vi "Document VI.vi"(6 "Variant in":variant, 7 "Shift Pressed?":bool, 8 "error in (no error)":errorcluster, 10 "QD Combo Box Ref":refnum<vi>, 11 "QD Launch VI Ref":refnum<vi>) -> (0 "error out":errorcluster, 4 "Variant out":variant)   [LabVIEW 2020, in "lv_documentation.lvlib"]
doc: "Write a 1-2 sentence description of the functionality of your plugin here. Replace the \"$\" below with the character you wish to assign as the default shortcut for this plugin. Do not add any text after the 'Default Shortcut' line below.\n\nDefault Shortcut - [$]"
uses:
  lv_documentation.lvlib
panel:
  in  "Undo Name":string="Quick Drop Keyboard Shortcut"
  # "Specify the name of the Undo transaction"
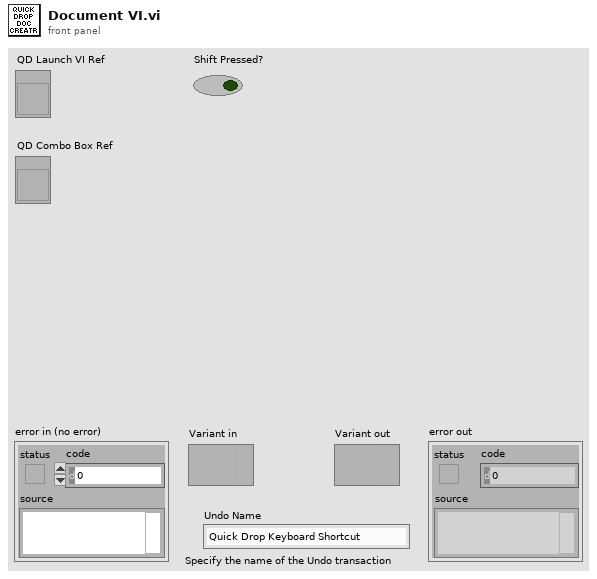
[diagram p1: front panel]
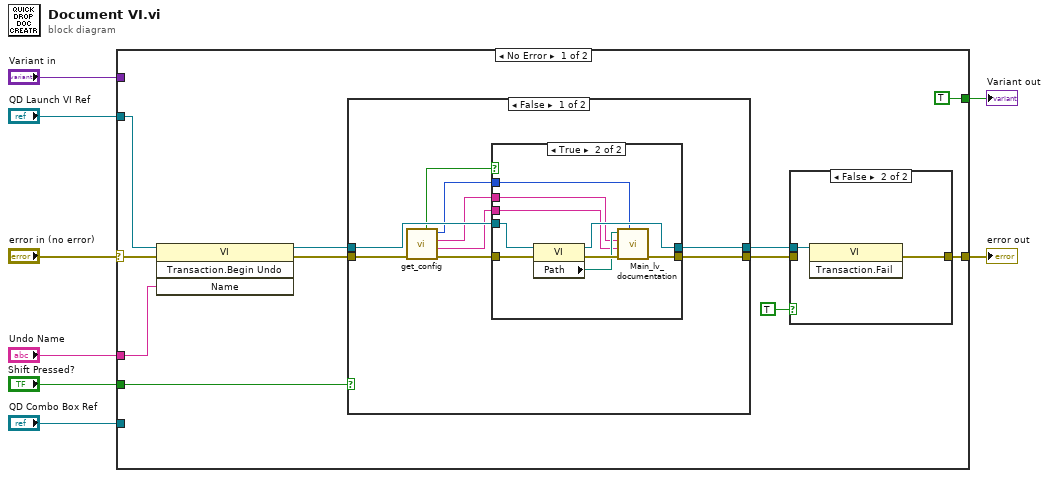
[diagram p0: block diagram]
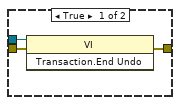
[diagram p2: hidden frame]
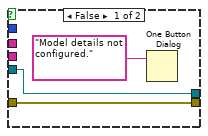
[diagram p3: hidden frame]
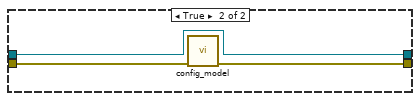
[diagram p4: hidden frame]
diagram:
  n1 = case shown="No Error" "error in (no error)" {
    selector: "error in (no error)" -> [w19 w49]
    tunnel: [w15 w49] -> w7
    tunnel: "QD Launch VI Ref" -> [w18 _]
    tunnel: "Shift Pressed?" -> [w9 _]
    tunnel: "QD Combo Box Ref" -> [_ _]
    tunnel: "Variant in" -> [_ _]
    tunnel: "Undo Name" -> [w17 _]
    tunnel: [TRUE _] -> w1
    frame No Error {
      n2 = invoke class="VI" method="Transaction.Begin Undo"(reference=w18, error in=w19, "Name"=w17) -> (reference out=w11:refnum<vi>, error out=w12:errorcluster)  [unwired: 1 in, 2 out]
      n3 = case shown="False" w9 {
        tunnel: [w33 w47] -> w13
        tunnel: w12 -> [w32 w48]
        tunnel: w11 -> [w31 w46]
        tunnel: [w30 w46] -> w10
        frame False {
          n4 = call "get_config.vi"("error in"=w32) -> ("error out"=w29:errorcluster, "key"=w25:string, "model name"=w27:string, "Provider Selector"=w26:enum32{"OpenAI", "Gemini"}, "proper config?"=w28:bool)  [unwired: 6 in]
          n5 = case shown="True" w28 {
            tunnel: [w36 w45] -> w33
            tunnel: w31 -> [w34 w42]
            tunnel: [w34 w41] -> w30
            tunnel: w29 -> [w36 w40]
            tunnel: w27 -> [_ w39]
            tunnel: w26 -> [_ w37]
            tunnel: w25 -> [_ w38]
            frame False {
              n6 = One Button Dialog(message="Model details not configured.") -> ()  [unwired: 1 in, 1 out]
            }
            frame True {
              n7 = property class="VI"(reference=w42, error in=w40) -> (reference out=w41:refnum<vi>, error out=w44:errorcluster, "Path"=w43:path)
              n8 = call "Main_lv_documentation.vi"("Provider Selector"=w37, "error in (no error)"=w44, "API Key"=w38, "model_name"=w39, "VI path"=w43) -> ("error out"=w45:errorcluster)  [unwired: 6 in]
            }
          }
        }
        frame True {
          n9 = call "config_model.vi"("error in (no error)"=w48) -> ("error out"=w47:errorcluster)  [unwired: 10 in]
        }
      }
      n10 = case shown="False" TRUE {
        tunnel: w10 -> [w21 w23]
        tunnel: [w22 w24] -> w15
        tunnel: w13 -> [w20 _]
        frame True {
          n11 = invoke class="VI" method="Transaction.End Undo"(reference=w21, error in=w20) -> (error out=w22:errorcluster)  [unwired: 1 in, 2 out]
        }
        frame False {
          n12 = invoke class="VI" method="Transaction.Fail"(reference=w23) -> (error out=w24:errorcluster)  [unwired: 2 in, 2 out]
        }
      }
    }
    frame Error {
    }
  }
  "error out" <- w7
  "Variant out" <- w1
